vi "_dealWithIndex_EEPROM_vna_wmg.vi"(0 "index":i32[](array[numeric])=[1, 2, 3, 5, 6, 7, 11, 12]) -> (1 "str":string, 2 "Flag":i32[][](array[numeric]))   [LabVIEW 2011]
panel:
  out "flag_b":i32
  out "flag_e":i32
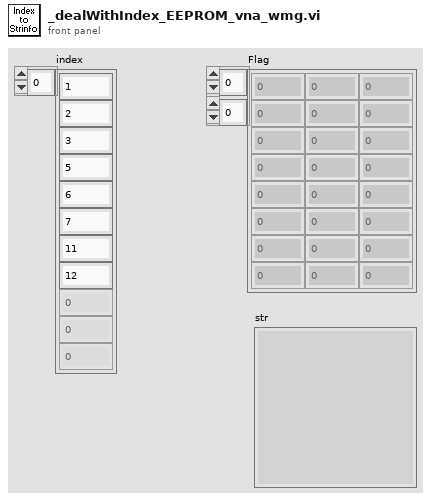
[diagram p1: front panel]
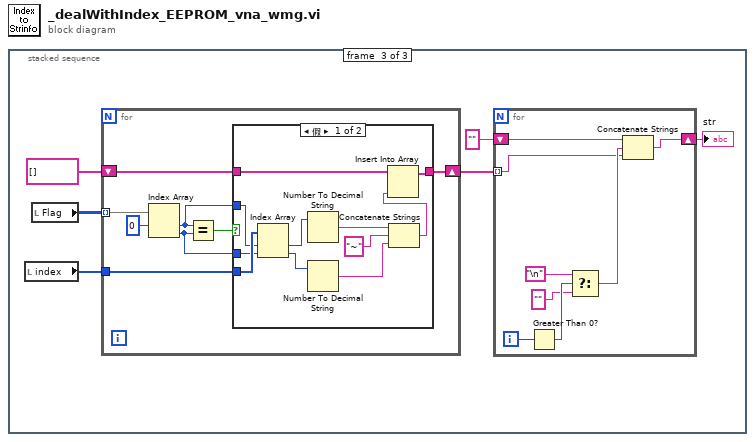
[diagram p0: block diagram]
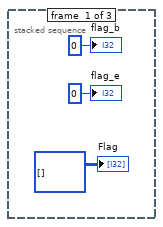
[diagram p2: hidden frame]
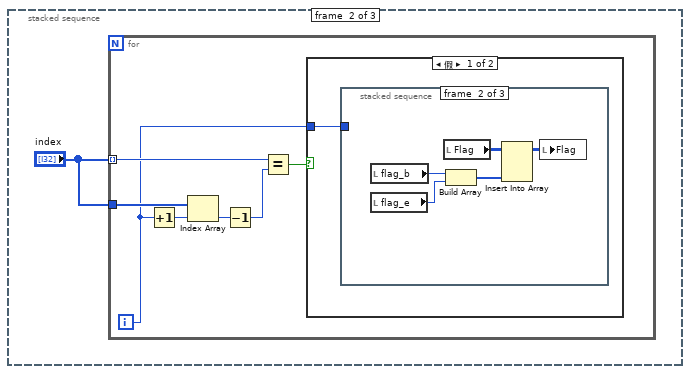
[diagram p3: hidden frame]
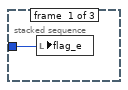
[diagram p4: hidden frame]
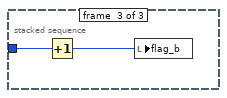
[diagram p5: hidden frame]
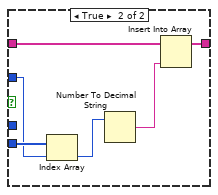
[diagram p7: hidden frame]
diagram:
  n1 = stacked-sequence {
    frame #0 {
      "flag_e" <- 0 ("flag")
      "Flag" <- i32[][] [] ("Flag")
      "flag_b" <- 0 ("flag 2")
    }
    frame #1 {
      n2 = for {
        tunnel: "index" -> [w6] mode=indexing
        tunnel: "index" -> [w11]
        i -> [w5]
        n3 = Increment(x=w5) -> (x+1=w10:i32)
        n4 = Index Array(array=w11, index=w10) -> (element=w9:i32)
        n5 = Decrement(x=w9) -> (x-1=w8:i32)
        n6 = Equal?(x=w6, y=w8) -> (x = y?=w7:bool)
        n7 = case shown="假" w7 {
          tunnel: w5 -> [w12 _]
          frame False {
            n8 = stacked-sequence {
              tunnel: w12 -> [w13 _ w20]
              frame #0 {
                n9 = local write "flag_e"(w13) -> ()
              }
              frame #1 {
                n10 = local read "flag_b"() -> (w15:i32)
                n11 = local read "flag_e"() -> (w14:i32)
                n12 = local read "Flag"() -> (w18:i32[][])
                n13 = Build Array(w15, w14) -> (w17:i32[])
                n14 = Insert Into Array(array=w18, new element=w17) -> (w16:i32[][])  [unwired: 2 in]
                n15 = local write "Flag"(w16) -> ()
              }
              frame #2 {
                n16 = Increment(x=w20) -> (x+1=w19:i32)
                n17 = local write "flag_b"(w19) -> ()
              }
            }
          }
          frame True {
          }
        }
      }
    }
    frame #2 {
      n18 = local read "index"() -> (w21:i32[])
      n19 = local read "Flag"() -> (w26:i32[][])
      n20 = for {
        tunnel: w26 -> [w42] mode=indexing
        shift-right: [w37] -> w24
        shift-left: string[] [] -> [w39]
        tunnel: w21 -> [w35]
        n21 = Index Array(array=w42, index #1=0 ("索引")) -> (element #1=w38:i32, element #2=w36:i32)  [unwired: 1 in]
        n22 = Equal?(x=w38, y=w36) -> (x = y?=w40:bool)
        n23 = case shown="假" w40 {
          tunnel: w39 -> [w53 w59]
          tunnel: w38 -> [w46 w55]
          tunnel: [w52 w57] -> w37
          tunnel: w36 -> [w45 _]
          tunnel: w35 -> [w47 w56]
          frame False {
            n24 = Index Array(array=w47, index #1=w46, index #2=w45) -> (element #1=w44:i32, element #2=w43:i32)
            n25 = Number To Decimal String(number=w44) -> (decimal integer string=w51:string)  [unwired: 1 in]
            n26 = Number To Decimal String(number=w43) -> (decimal integer string=w49:string)  [unwired: 1 in]
            n27 = Concatenate Strings(w51, "~", w49) -> (w48:string)
            n28 = Insert Into Array(array=w53, new element=w48) -> (w52:string[])  [unwired: 1 in]
          }
          frame True {
            n29 = Index Array(array=w56, index=w55) -> (element=w54:i32)
            n30 = Number To Decimal String(number=w54) -> (decimal integer string=w58:string)  [unwired: 1 in]
            n31 = Insert Into Array(array=w59, new element=w58) -> (w57:string[])  [unwired: 1 in]
          }
        }
      }
      n32 = for {
        tunnel: w24 -> [w28] mode=indexing
        shift-right: [w27] -> w22
        shift-left: "" -> [w30]
        i -> [w34]
        n33 = Greater Than 0?(x=w34) -> (x > 0?=w33:bool)
        n34 = Select(t="\n", s=w33, f="") -> (s? t:f=w29:string)
        n35 = Concatenate Strings(w30, w29, w28) -> (w27:string)
      }
      "str" <- w22
    }
  }
